vi "Remove Handler.vi"(8 "error in":errorcluster, 10 "Name":string, 11 "Logger in":refnum<class "Logger.lvclass">) -> (0 "error out":errorcluster, 3 "Logger out":refnum<class "Logger.lvclass">)   [LabVIEW 2020, in "hse-logger.lvlib" / "Logger.lvclass"]
doc: "Removes a handler specified by ``Name``. \nIf there is no handler with the searched name, nothing is removed and rais an error \"510802 - Handler name not found\".\n\n____\nHAMPEL SOFTWARE ENGINEERING v2.0.6 (2021-04-15 11:38)"
uses:
  Logger.lvclass
  Logger.lvclass/Logger.ctl
  Handler/Handler.lvclass
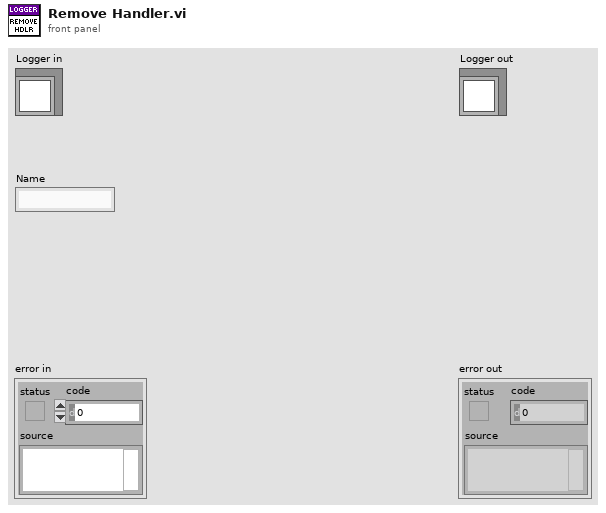
[diagram p1: front panel]
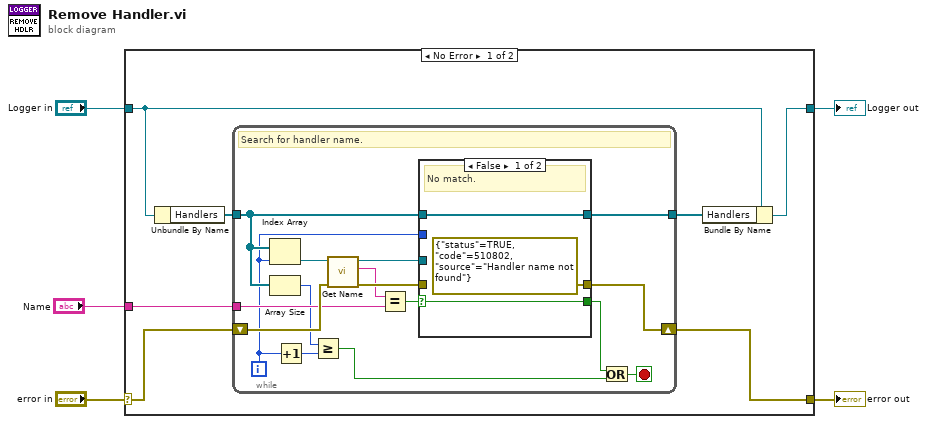
[diagram p0: block diagram]
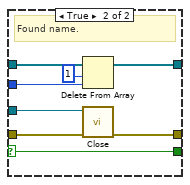
[diagram p2: hidden frame]
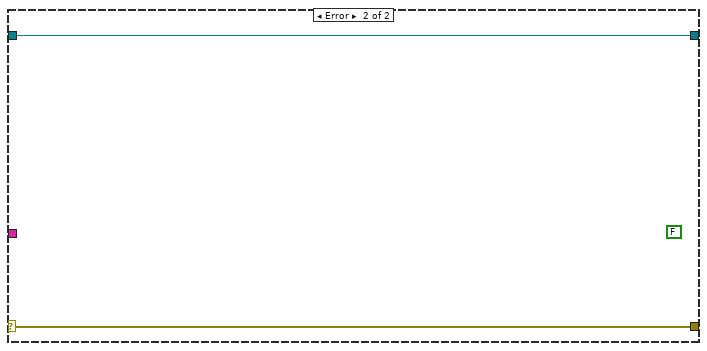
[diagram p3: hidden frame]
diagram:
  n1 = case shown="No Error" "error in" {
    selector: "error in" -> [w11 w41]
    tunnel: [w6 w41] -> w4
    tunnel: [w8 w40] -> w2
    tunnel: "Logger in" -> [w9 w40]
    tunnel: "Name" -> [w10 _]
    frame No Error {
      n2 = Unbundle By Name(w9) -> ("Handlers"=w12:refnum<class "Handler.lvclass">[])
      n3 = while {
        tunnel: w12 -> [w17]
        shift-right: [w22] -> w6
        shift-left: w11 -> [w27]
        tunnel: w10 -> [w26]
        tunnel: [w15] -> w7
        i -> [w16]
        stop <- w19 stop-if-true
        # "Search for handler name."
        n4 = Index Array(array=w17, index=w16) -> (element=w21:refnum<class "Handler.lvclass">)
        n5 = Array Size(array=w17) -> (size(s)=w20:i32)
        n6 = Increment(x=w16) -> (x+1=w14:i32)
        n7 = Greater Or Equal?(x=w20, y=w14) -> (x >= y?=w18:bool)
        n8 = call-dynamic "Get Name.vi"("error in"=w27, "Handler in"=w21) -> ("error out"=w28:errorcluster, "Name"=w25:string, "Handler out"=w23:refnum<class "Handler.lvclass">)  [unwired: 7 in]
        n9 = Equal?(x=w25, y=w26) -> (x = y?=w24:bool)
        n10 = case shown="False" w24 {
          selector: w24 -> [w30 w32]
          tunnel: w28 -> [_ w38]
          tunnel: w23 -> [_ w39]
          tunnel: [w30 w32] -> w13
          tunnel: [errorcluster {"status"=TRUE, "code"=510802, "source"="Handler name not found"} ("error out") w37] -> w22
          tunnel: w17 -> [w31 w36]
          tunnel: w16 -> [_ w34]
          tunnel: [w31 w33] -> w15
          frame False {
            # "No match."
          }
          frame True {
            # "Found name."
            n11 = Delete From Array(array=w36, length=1, index=w34) -> (array with subset deleted=w33:refnum<class "Handler.lvclass">[])  [unwired: 1 out]
            n12 = call-dynamic "Close.vi"("error in"=w38, "Handler in"=w39) -> ("error out"=w37:errorcluster)  [unwired: 8 in, 1 out]
          }
        }
        n13 = Or(x=w13, y=w18) -> (x .or. y?=w19:bool)
      }
      n14 = Bundle By Name(cluster=w9, "Handlers"=w7) -> (w8:refnum<class "Logger.lvclass">)
    }
    frame Error {
      (unwired) FALSE
    }
  }
  "error out" <- w4
  "Logger out" <- w2
